vi "Autonomous Independent.vi"   [LabVIEW 2019]
doc: "This VI is called when autonomous begins, and will automatically be terminated when autonomous ends. You can carry out timed or sensor driven robot movement independently without needing to return to the caller."
uses:
  <vilib>/Rock Robotics/Network Tables/NT Read String.vi
  Drive/Drive Global.vi
  Shoot/Shoot Global.vi
  Intake/Intake Global.vi
  Index/Index Global.vi
panel:
  # "Be sure to right-click and choose Data Operations>>Make Current Value default if you want to save the array values with the VI"
types:
  T1 = typedef "Auton Subsystems Steps Typedef.ctl" = cluster{"Drive Command":T2, "Shoot Auton Command":T4, "Intake Command":T7, "Index Motor Values":dbl, "Max time to complete step (ms)":dbl, "Min. Time to complete step (ms)":dbl}
  T2 = typedef "Drive Command Typedef.ctl" = cluster{"Drive Mode":T3, "LeftValue(%)/ relative Distance[ft]":dbl, "Right Motor Value(%)/ absolute angle (deg)":dbl, "Timestamp (ms)":dbl}
  T3 = typedef "Drive Mode Typedef.ctl" = enum16{"Disabled", "Auto-align", "Drive Distance", "Turn to angle", "Driver"}
  T4 = typedef "Shooter Command Type Def.ctl" = cluster{"Shooter Mode":T5, "Throttle (%)/ Vision-based\nSetpoint (RPM)":dbl, "Shooter Preset speeds (RPM)":T6, "Timestamp (ms)":dbl}
  T5 = typedef "Shooter Mode Type Def.ctl" = enum16{"Disabled", "Raw Throttle", "Preset Velocity Control", "Vision-based Velocity Control"}
  T6 = typedef "Shooter Preset speeds Type Def.ctl" = enum16{"Not Applicable", "Target Zone", "Initiation Line", "Close end of Trench Run", "Control Panel"}
  T7 = typedef "Intake Command Type Def.ctl" = cluster{"Intake Mode":T8, "Throttle (%)":dbl, "Pneumatic State":T9}
  T8 = typedef "Intake Mode Type Def.ctl" = enum16{"Disabled", "Enabled"}
  T9 = typedef "WPI_SolenoidValue.ctl" = enum16{"Off", "On", "Forward", "Reverse"}
  T10 = typedef "Is command done typedef.ctl" = cluster{"Done?":bool, "Timestamp [ms]":dbl}
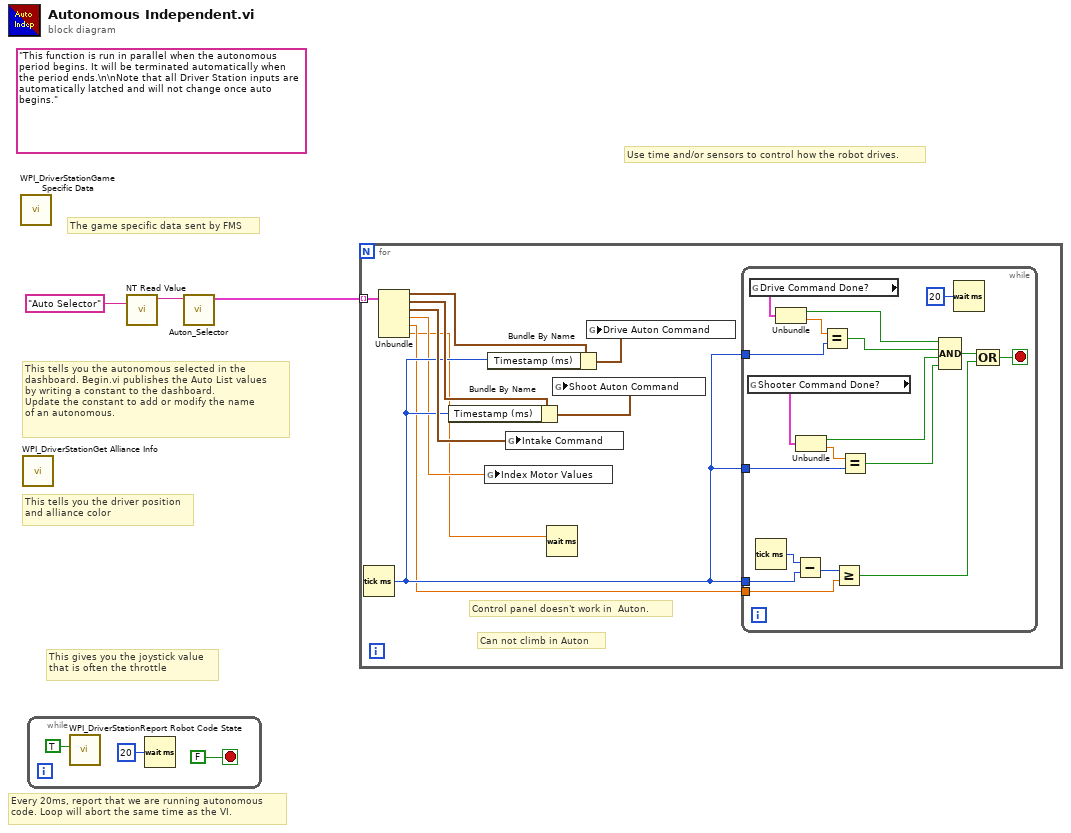
[diagram p0: block diagram]
diagram:
  (unwired) "This function is run in parallel when the autonomous period begins. It will be terminated automatically when the period ends.\n\nNote that all Driver Station inputs are automatically latched and will not change once auto begins."
  # "The game specific data sent by FMS"
  # "This tells you the autonomous selected in the \ndashboard. Begin.vi publishes the Auto List values\nby writing a constant to the dashboard.\nUpdate the constant to add or modify the name\nof an autonomous."
  # "Every 20ms, report that we are running autonomous\ncode. Loop will abort the same time as the VI."
  # "This gives you the joystick value\nthat is often the throttle"
  # "Use time and/or sensors to control how the robot drives."
  # "This tells you the driver position\nand alliance color"
  n1 = call <vilib>:"WPI_DriverStationGame Specific Data.vi"() -> ()  [unwired: 11 in, 1 out]
  n2 = call <vilib>:"WPI_DriverStationGet Alliance Info.vi"() -> ()  [unwired: 12 out]
  n3 = while {
    stop <- FALSE stop-if-true
    n4 = call <vilib>:"WPI_DriverStationReport Robot Code State.vi"("Autonomous"=TRUE) -> ()  [unwired: 10 in, 1 out]
    n5 = Wait (ms)(milliseconds to wait=u32 20) -> ()  [unwired: 1 out]
  }
  n6 = call-poly <vilib>:"NT Read Value.vi"("Name"="Auto Selector") -> ("String"=w2:string)  [unwired: 9 in, 1 out]
  n7 = call "Auton_Selector.vi"("Auton Name In"=w2) -> ("Auton Steps"=w1:T1[])  [unwired: 10 in]
  n8 = for {
    tunnel: w1 -> [w16] mode=indexing
    # "Can not climb in Auton"
    # "Control panel doesn't work in  Auton."
    n9 = Tick Count (ms)() -> (millisecond timer value=w10:u32)
    n10 = Unbundle(w16) -> ("Drive Command"=w14:T2, "Shoot Auton Command"=w13:T4, "Intake Command"=w11:T7, "Index Motor Values"=w9:dbl, "Max time to complete step (ms)"=w8:dbl, "Min. Time to complete step (ms)"=w7:dbl)
    n11 = Bundle By Name(cluster=w13, "Timestamp (ms)"=w10) -> (w12:T4)
    n12 = global write "Index Global.vi" "Index Motor Values"(w9) -> ()
    n13 = Bundle By Name(cluster=w14, "Timestamp (ms)"=w10) -> (w15:T2)
    n14 = global write "Intake Global.vi" "Intake Command"(w11) -> ()
    n15 = Wait (ms)(milliseconds to wait=w7) -> ()  [unwired: 1 out]
    n16 = global write "Shoot Global.vi" "Shoot Auton Command"(w12) -> ()
    n17 = global write "Drive Global.vi" "Drive Auton Command"(w15) -> ()
    n18 = while {
      tunnel: w10 -> [w28]
      tunnel: w10 -> [w32]
      tunnel: w10 -> [w21]
      tunnel: w8 -> [w17]
      stop <- w30 stop-if-true
      n19 = global read "Shoot Global.vi" "Shooter Command Done?"() -> (w18:T10)
      n20 = global read "Drive Global.vi" "Drive Command Done?"() -> (w19:T10)
      n21 = Tick Count (ms)() -> (millisecond timer value=w33:u32)
      n22 = Unbundle(w19) -> ("Done?"=w26:bool, "Timestamp [ms]"=w27:dbl)
      n23 = Subtract(x=w33, y=w32) -> (x-y=w31:u32)
      n24 = Unbundle(w18) -> ("Done?"=w23:bool, "Timestamp [ms]"=w22:dbl)
      n25 = Equal?(x=w27, y=w28) -> (x = y?=w25:bool)
      n26 = Greater Or Equal?(x=w31, y=w17) -> (x >= y?=w24:bool)
      n27 = Equal?(x=w22, y=w21) -> (x = y?=w20:bool)
      n28 = Compound Arithmetic op=AND(w26, w25, w23, w20) -> (w29:bool)
      n29 = Wait (ms)(milliseconds to wait=u32 20) -> ()  [unwired: 1 out]
      n30 = Compound Arithmetic op=OR(w29, w24) -> (w30:bool)
    }
  }
